vi "main002.vi"() -> ()   [LabVIEW 2019]
uses:
  <vilib>/DAQmx/write.llb/DAQmx Write (Analog DBL 1Chan 1Samp).vi
  <vilib>/DAQmx/miscellaneous.llb/DAQmx Fill In Error Info.vi
  <vilib>/DAQmx/create/channels.llb/DAQmx Create Channel (AO-Voltage-Basic).vi
  libs/Newport ESP301/Newport ESP301.lvlib
panel:
  in  "Boolean":bool
  out "a":waveform(dbl)(graph)={"t0"=timestamp(3633530059.5453157 s since 1904-01-01), "dt"=1.0, "Y"=[nan]}
  out "Waveform Chart":dbl(graph)=5.25341140860948
  out "x*y":dbl=nan
  in  "physical channels":tag="Dev3/ao1"
  out "DAC error":errorcluster
  out "ESP error":errorcluster={"status"=TRUE, "code"=-1074000000, "source"="Newport ESP301.lvlib:Error Query.vi<ERR>\nInstrument reports:\n313, 62119445, AXIS-3 MOTOR NOT ENABLED\r\n313, 62124900, AXIS-3 MOTOR NOT ENABLED\r\n313, 62130330, AXIS-3 MOTOR NOT ENABLED\r\n313, 62135785, AXIS-3 MOTOR NOT ENABLED\r\n313, 62141219, AXIS-3 MOTOR NOT ENABLED\r\n313, 62146768, AXIS-3 MOTOR NOT ENABLED\r\n313, 62152226, AXIS-3 MOTOR NOT ENABLED\r\n313, 62157684, AXIS-3 MOTOR NOT ENABLED\r\n313, 62163236, AXIS-3 MOTOR NOT ENABLED\r\n313, 62168690, AXIS-3 MOTOR NOT ENABLED\r\n0, 499821715, NO ERROR DETECTED\r\n\n\n\n<b>Complete call chain:</b>\r\n     Newport ESP301.lvlib:Error Query.vi\r\n     Newport ESP301.lvlib:Initialize.vi\r\n     main002.vi"}
  out "run?":bool
  in  "set_vel":bool
  in  "velocity [fs/s]":dbl=667.128190396304
  in  "vel_mm":dbl caption="velocity [mm/s]"
  out "meas. velocity":dbl=nan
  in  "stop":bool
  out "output voltage":dbl=nan
  in  "start":bool
  in  "go2p1":bool
  out "position [fs]":dbl=nan
  out "position [mm]":dbl=nan
  in  "p2 [mm]":dbl=2.0
  in  "p1 [mm]":dbl
  in  "interpolate output":bool
  in  "t2 [fs]":dbl=6671.281903963041
  in  "t1 [fs]":dbl=-6671.281903963041
  in  "t0 [mm]":dbl=1.0
  in  "Axis (1)":i32=3 min=1 max=3
  in  "Serial Link (RS232)":enum16{"RS232", "USB"}(ring)
  in  "VISA resource name":refnum<visa-resource-name>="COM9"
  in  "main_close":bool
  # "Always use CLOSE button to correctly disconnect the device. STOP program afterwards."
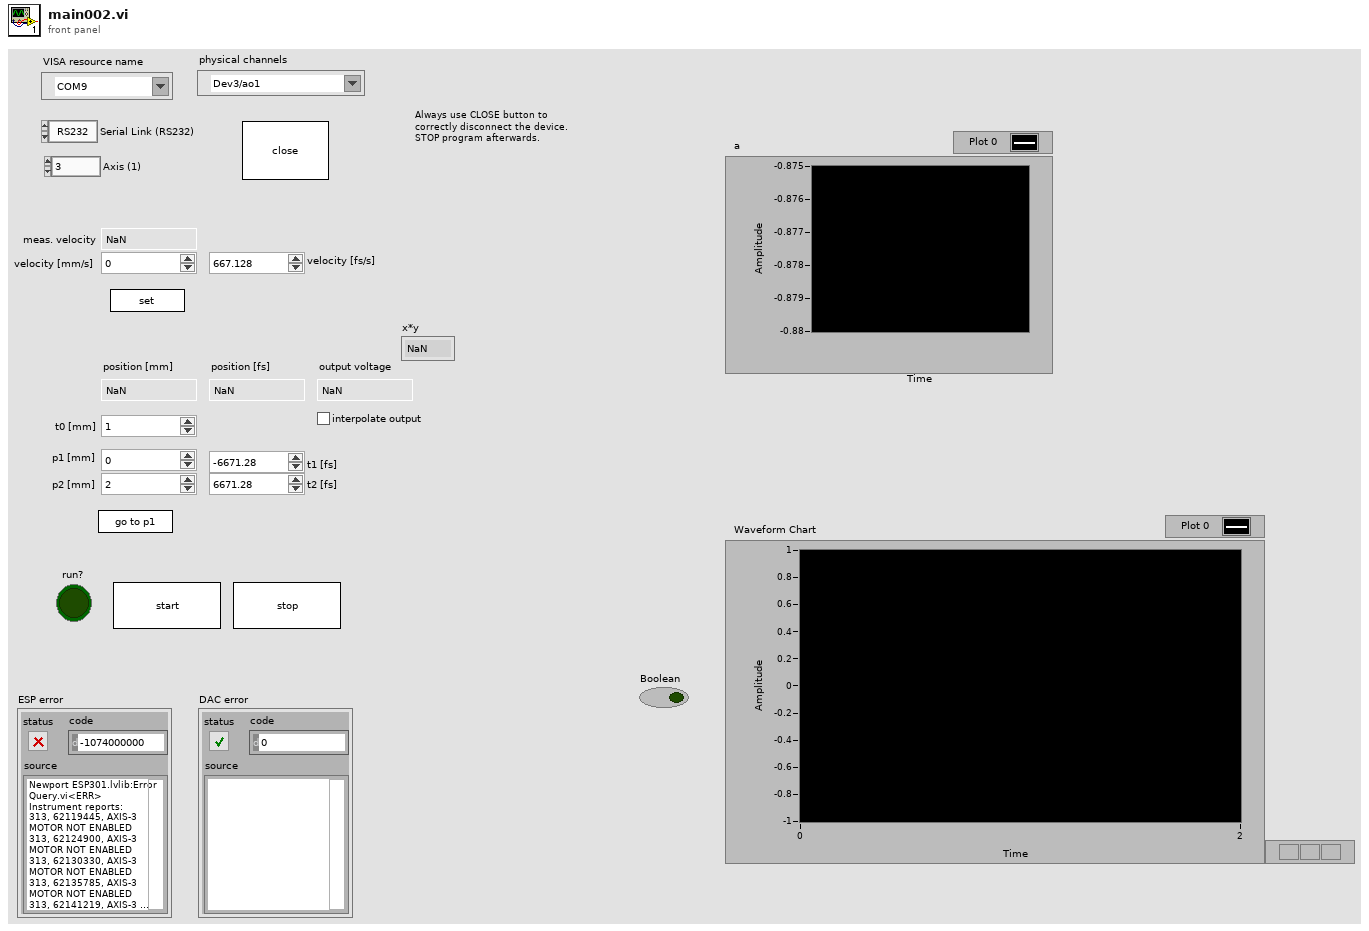
[diagram p1: front panel]
types:
  T1 = cluster{"dev1_data":refnum<queue>, "dev2_data":refnum<queue>}
  T2 = cluster{"dev1_cmd":refnum<queue>, "dev2_cmd":refnum<queue>}
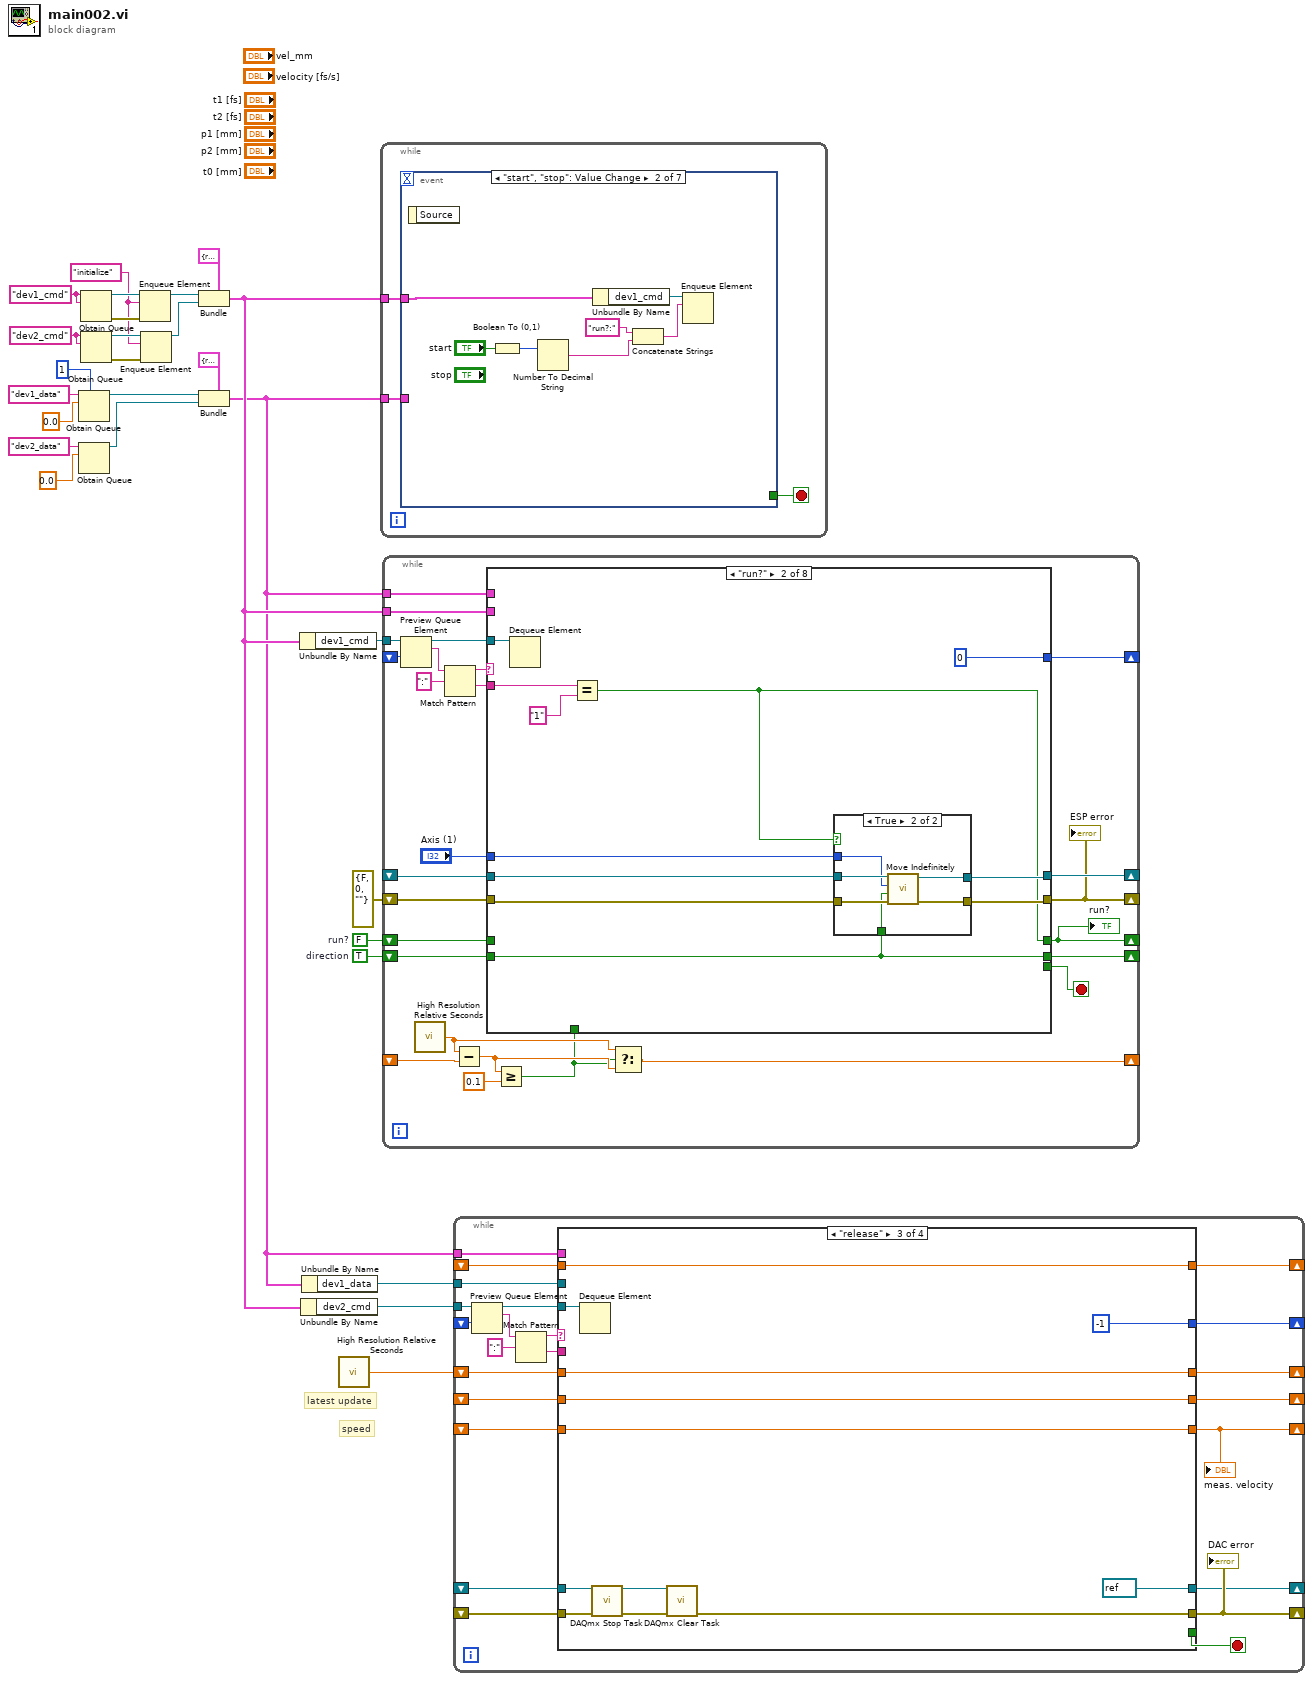
[diagram p0: block diagram]
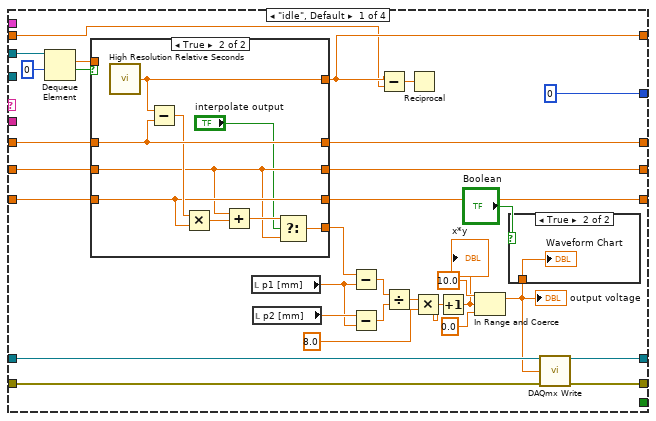
[diagram p2: hidden frame]
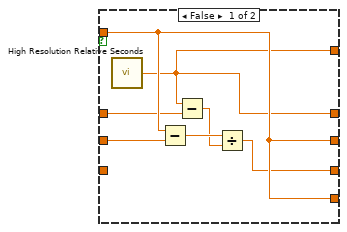
[diagram p4: hidden frame]
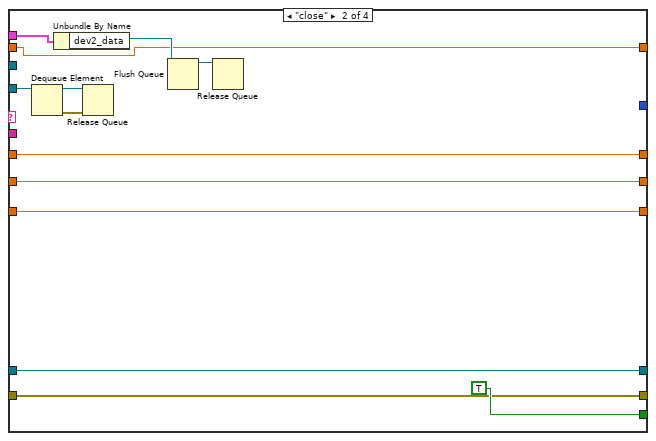
[diagram p5: hidden frame]
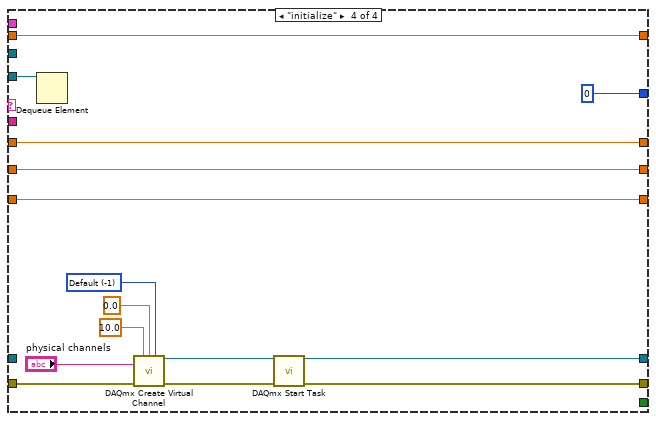
[diagram p6: hidden frame]
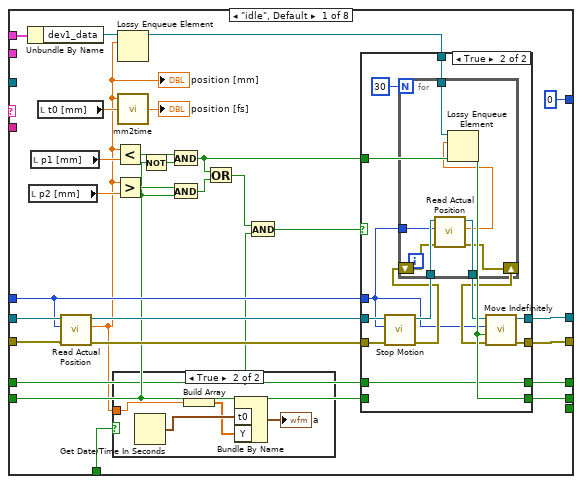
[diagram p7: hidden frame]
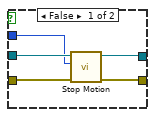
[diagram p10: hidden frame]
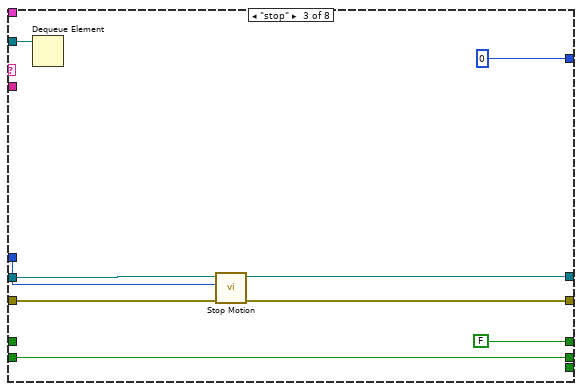
[diagram p11: hidden frame]
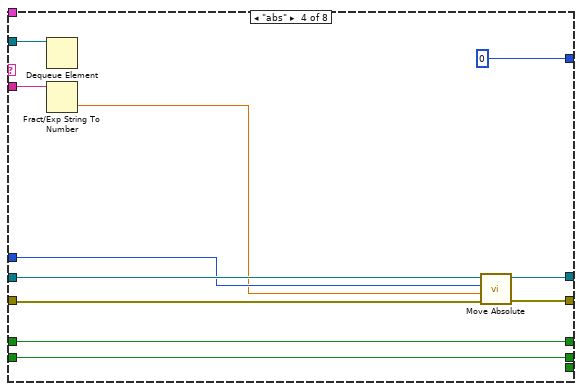
[diagram p12: hidden frame]
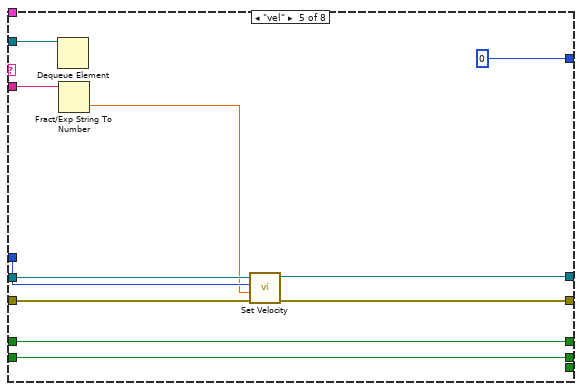
[diagram p13: hidden frame]
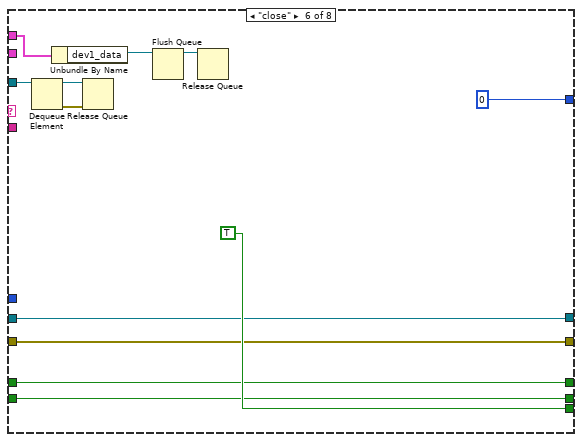
[diagram p14: hidden frame]
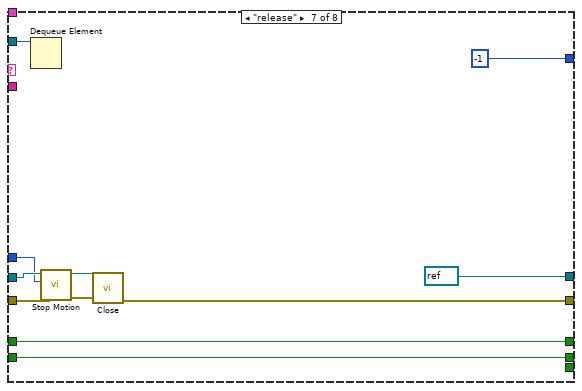
[diagram p15: hidden frame]
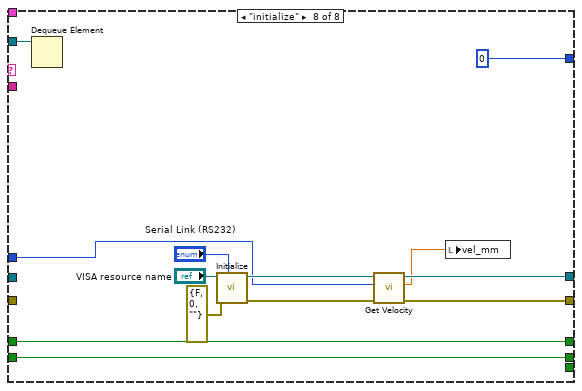
[diagram p16: hidden frame]
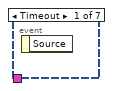
[diagram p17: hidden frame]
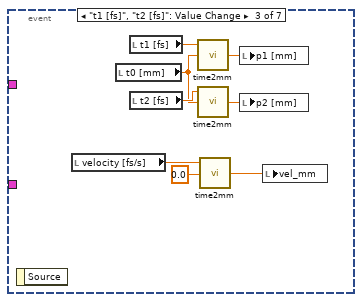
[diagram p18: hidden frame]
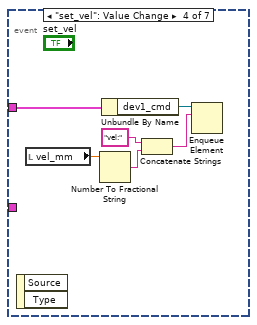
[diagram p19: hidden frame]
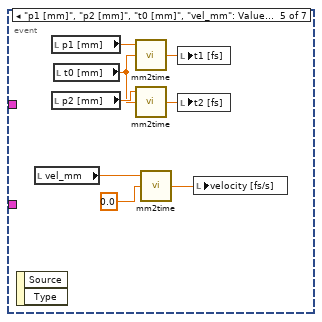
[diagram p20: hidden frame]
diagram:
  w1 = TRUE  # direction
  w4 = FALSE  # run?
  w15 = "dev2_cmd" ("name (unnamed)")
  w21 = "initialize" ("element")
  w16 = "dev1_cmd" ("name (unnamed)")
  # "speed"
  # "latest update"
  n1 = Obtain Queue(max queue size (-1, unlimited)=1, name (unnamed)="dev1_data", element data type=0.0) -> (queue out=w12:refnum<queue>)  [unwired: 2 in, 2 out]
  n2 = Obtain Queue(name (unnamed)="dev2_data", element data type=0.0) -> (queue out=w11:refnum<queue>)  [unwired: 3 in, 2 out]
  n3 = Obtain Queue(name (unnamed)=w16, element data type=w16) -> (queue out=w27:refnum<queue>, error out=w26:errorcluster)  [unwired: 3 in, 1 out]
  n4 = Obtain Queue(name (unnamed)=w15, element data type=w15) -> (queue out=w22:refnum<queue>, error out=w23:errorcluster)  [unwired: 3 in, 1 out]
  n5 = Enqueue Element(queue=w27, element=w21, error in (no error)=w26) -> (queue out=w24:refnum<queue>)  [unwired: 1 in, 2 out]
  n6 = Enqueue Element(queue=w22, element=w21, error in (no error)=w23) -> (queue out=w20:refnum<queue>)  [unwired: 1 in, 2 out]
  n7 = Bundle(cluster=T2 {"dev1_cmd"=refnum, "dev2_cmd"=refnum}, "dev1_cmd"=w24, "dev2_cmd"=w20) -> (w8:T2)
  n8 = Bundle(cluster=T1 {"dev1_data"=refnum, "dev2_data"=refnum}, "dev1_data"=w12, "dev2_data"=w11) -> (w2:T1)
  n9 = Unbundle By Name(w8) -> ("dev1_cmd"=w17:refnum<queue>)
  n10 = Unbundle By Name(w8) -> ("dev2_cmd"=w7:refnum<queue>)
  n11 = Unbundle By Name(w2) -> ("dev1_data"=w6:refnum<queue>)
  n12 = call <vilib>:"High Resolution Relative Seconds.vi"() -> ("relative seconds"=w5:dbl)
  n13 = while {
    tunnel: w8 -> [w30]
    tunnel: w2 -> [w29]
    stop <- w28 stop-if-true
    n14 = event shown="[1] \"start\", \"stop\": Value Change" {
      selector: _ -> [_ _ _ _ _ _ _]
      dyn-events: _ -> [_ _ _ _ _ _ _]
      timeout: _ -> [_ _ _ _ _ _ _]
      tunnel: w30 -> [_ w34 _ w47 _ w65 w68]
      tunnel: w29 -> [_ _ _ _ _ _ _]
      tunnel: [_ _ _ _ _ _ TRUE] -> w28
      event Timeout {
        n15 = event-data() -> ()  [unwired: 1 in, 1 out]
      }
      event "start", "stop": Value Change {
        n16 = event-data() -> ()  [unwired: 1 in, 1 out]
        n17 = Boolean To (0,1)(Boolean="start") -> (0, 1=w32:i16)
        n18 = Number To Decimal String(number=w32) -> (decimal integer string=w31:string)  [unwired: 1 in]
        n19 = Unbundle By Name(w34) -> ("dev1_cmd"=w37:refnum<queue>)
        n20 = Concatenate Strings("run?:" ("string"), w31) -> (w36:string)
        n21 = Enqueue Element(queue=w37, element=w36) -> ()  [unwired: 2 in, 3 out]
      }
      event "t1 [fs]", "t2 [fs]": Value Change {
        n22 = event-data() -> ()  [unwired: 1 in, 1 out]
        n23 = local read "velocity [fs/s]"() -> (w40:dbl)
        n24 = local read "t0 [mm]"() -> (w43:dbl)
        n25 = local read "t1 [fs]"() -> (w44:dbl)
        n26 = local read "t2 [fs]"() -> (w45:dbl)
        n27 = call "time2mm.vi"("Offset (mm)"=w43, "time"=w44) -> ("position (mm)"=w41:dbl)  [unwired: 1 in]
        n28 = call "time2mm.vi"("Offset (mm)"=w43, "time"=w45) -> ("position (mm)"=w42:dbl)  [unwired: 1 in]
        n29 = call "time2mm.vi"("Offset (mm)"=0.0, "time"=w40) -> ("position (mm)"=w38:dbl)  [unwired: 1 in]
        n30 = local write "p1 [mm]"(w41) -> ()
        n31 = local write "p2 [mm]"(w42) -> ()
        n32 = local write "vel_mm"(w38) -> ()
      }
      event "set_vel": Value Change {
        n33 = event-data() -> ()  [unwired: 1 in, 2 out]
        n34 = local read "vel_mm"() -> (w46:dbl)
        n35 = Number To Fractional String(number=w46) -> (F-format string=w50:string)  [unwired: 3 in]
        n36 = Unbundle By Name(w47) -> ("dev1_cmd"=w51:refnum<queue>)
        n37 = Concatenate Strings("vel:" ("string"), w50) -> (w49:string)
        n38 = Enqueue Element(queue=w51, element=w49) -> ()  [unwired: 2 in, 3 out]
      }
      event "p1 [mm]", "p2 [mm]", "t0 [mm]", "vel_mm": Value Change {
        n39 = event-data() -> ()  [unwired: 1 in, 2 out]
        n40 = local read "vel_mm"() -> (w54:dbl)
        n41 = local read "p1 [mm]"() -> (w58:dbl)
        n42 = local read "p2 [mm]"() -> (w59:dbl)
        n43 = local read "t0 [mm]"() -> (w57:dbl)
        n44 = call "mm2time.vi"("Offset (mm)"=w57, "distance (mm)"=w58) -> ("time in fs"=w55:dbl)  [unwired: 1 in]
        n45 = call "mm2time.vi"("Offset (mm)"=w57, "distance (mm)"=w59) -> ("time in fs"=w56:dbl)  [unwired: 1 in]
        n46 = call "mm2time.vi"("Offset (mm)"=0.0, "distance (mm)"=w54) -> ("time in fs"=w53:dbl)  [unwired: 1 in]
        n47 = local write "t1 [fs]"(w55) -> ()
        n48 = local write "t2 [fs]"(w56) -> ()
        n49 = local write "velocity [fs/s]"(w53) -> ()
      }
      event "go2p1": Value Change {
        n50 = event-data() -> ()  [unwired: 1 in, 2 out]
        n51 = local read "p1 [mm]"() -> (w60:dbl)
        n52 = Number To Fractional String(number=w60) -> (F-format string=w63:string)  [unwired: 3 in]
        n53 = Unbundle By Name(w65) -> ("dev1_cmd"=w64:refnum<queue>)
        n54 = Concatenate Strings("abs:" ("string"), w63) -> (w61:string)
        n55 = Enqueue Element(queue=w64, element=w61) -> ()  [unwired: 2 in, 3 out]
      }
      event "main_close": Value Change {
        n56 = event-data() -> ()  [unwired: 1 in, 1 out]
        n57 = Cluster To Array(cluster=w68) -> (array=w67:refnum<queue>[])
        n58 = for {
          tunnel: w67 -> [w73] mode=indexing
          n59 = Flush Queue(queue=w73) -> (queue out=w69:refnum<queue>)  [unwired: 1 in, 2 out]
          n60 = Enqueue Element(queue=w69, element="release") -> (queue out=w71:refnum<queue>)  [unwired: 2 in, 2 out]
          n61 = Enqueue Element(queue=w71, element="close") -> ()  [unwired: 2 in, 3 out]
        }
      }
    }
  }
  n62 = while {
    tunnel: w8 -> [w94]
    tunnel: w17 -> [w99]
    tunnel: w2 -> [w91]
    shift-right: [w89] -> _
    shift-left: _ -> [w90]
    shift-right: [w88] -> _
    shift-left: _ -> [w85]
    shift-right: [w87] -> _
    shift-left: errorcluster {"status"=FALSE, "code"=0, "source"=""} ("error out") -> [w86]
    shift-right: [w82] -> _
    shift-left: w4 -> [w83]
    shift-right: [w80] -> _
    shift-left: w1 -> [w81]
    shift-right: [w74] -> _
    shift-left: _ -> [w79]
    stop <- w92 stop-if-true
    n63 = Preview Queue Element(queue=w99, timeout in ms (-1)=w90) -> (queue out=w93:refnum<queue>, element=w98:string)  [unwired: 1 in, 2 out]
    n64 = call <vilib>:"High Resolution Relative Seconds.vi"() -> ("relative seconds"=w76:dbl)
    n65 = Match Pattern(string=w98, regular expression=":") -> (before substring=w96:string, after substring=w95:string)  [unwired: 1 in, 2 out]
    n66 = Subtract(x=w76, y=w79) -> (x-y=w77:dbl)
    n67 = Greater Or Equal?(x=w77, y=0.1) -> (x >= y?=w75:bool)
    n68 = case shown="\"run?\"" w96 {
      tunnel: w95 -> [_ w166 _ w196 w203 _ _ _]
      tunnel: w94 -> [_ _ _ _ _ _ _ _]
      tunnel: w93 -> [_ w164 w179 w197 w201 w220 w230 w240]
      tunnel: [_ _ _ _ _ TRUE _ _] -> w92
      tunnel: w91 -> [w126 _ _ _ _ w212 _ _]
      tunnel: [0 0 0 0 0 0 -1 0] -> w89
      tunnel: [w122 w161 w184 w193 w208 w216 refnum<visa-resource-name> refnum ("VISA resource name out") w236] -> w88
      tunnel: [w121 w160 w183 w192 w207 w215 w229 w235] -> w87
      tunnel: w86 -> [w117 w158 w185 w194 w206 w215 w225 _]
      tunnel: w85 -> [w119 w159 w186 w195 w205 w216 w222 _]
      tunnel: "Axis (1)" -> [w118 w162 w182 w191 w204 _ w221 w237]
      tunnel: w83 -> [w104 _ _ w188 w199 w213 w227 w241]
      tunnel: [w103 w157 FALSE ("run?") w188 w199 w213 w227 w241] -> w82
      tunnel: w81 -> [w105 w156 w178 w187 w198 w209 w226 w232]
      tunnel: [w106 w156 w178 w187 w198 w209 w226 w232] -> w80
      tunnel: w75 -> [w102 _ _ _ _ _ _ _]
      frame "idle", Default {
        n69 = Unbundle By Name(w126) -> ("dev1_data"=w125:refnum<queue>)
        n70 = local read "p2 [mm]"() -> (w113:dbl)
        n71 = local read "p1 [mm]"() -> (w114:dbl)
        n72 = local read "t0 [mm]"() -> (w124:dbl)
        n73 = call "Read Actual Position.vi"("error in (no error)"=w117, "Axis (1)"=w118, "VISA resource name"=w119) -> ("error out"=w116:errorcluster, "Position (units)"=w101:dbl, "VISA resource name out"=w115:refnum<visa-resource-name>)  [unwired: 2 in]
        "position [mm]" <- w101
        n74 = case shown="True" w102 {
          tunnel: w101 -> [_ w131]
          frame False {
          }
          frame True {
            n75 = Get Date/Time In Seconds() -> (seconds since 1Jan1904=w130:timestamp)
            n76 = Build Array(w131) -> (w129:dbl[])
            n77 = Bundle By Name("t0"=w130, "Y"=w129) -> (→"a":waveform(dbl))  [unwired: 1 in]
          }
        }
        n78 = Less?(x=w101, y=w114) -> (x < y?=w111:bool)
        n79 = Greater?(x=w101, y=w113) -> (0:w110:bool)
        n80 = Lossy Enqueue Element(queue=w125, element=w101) -> (queue out=w100:refnum<queue>)  [unwired: 1 in, 3 out]
        n81 = call "mm2time.vi"("Offset (mm)"=w124, "distance (mm)"=w101) -> ("time in fs"=→"position [fs]":dbl)  [unwired: 1 in]
        n82 = Not(x=w105) -> (.not. x?=w112:bool)
        n83 = And(x=w111, y=w112) -> (x .and. y?=w107:bool)
        n84 = And(x=w110, y=w105) -> (x .and. y?=w109:bool)
        n85 = Or(x=w107, y=w109) -> (x .or. y?=w108:bool)
        n86 = And(x=w108, y=w104) -> (x .and. y?=w120:bool)
        n87 = case shown="True" w120 {
          tunnel: w115 -> [w135 w146]
          tunnel: w116 -> [w134 w145]
          tunnel: [w135 w148] -> w122
          tunnel: [w134 w147] -> w121
          tunnel: w118 -> [_ w138]
          tunnel: w107 -> [_ w144]
          tunnel: [w133 w144] -> w106
          tunnel: w105 -> [w133 _]
          tunnel: w104 -> [w132 w143]
          tunnel: [w132 w143] -> w103
          tunnel: w100 -> [_ w137]
          frame False {
          }
          frame True {
            n88 = call "Stop Motion.vi"("error in (no error)"=w145, "Axis (1)"=w138, "VISA resource name"=w146) -> ("error out"=w140:errorcluster, "VISA resource name out"=w142:refnum<visa-resource-name>)  [unwired: 3 in]
            n89 = for {
              N: 30 -> [_]
              tunnel: w142 -> [w155]
              tunnel: [w154] -> w141
              shift-right: [w152] -> w139
              shift-left: w140 -> [w153]
              tunnel: w138 -> [w151]
              tunnel: w137 -> [w150]
              n90 = call "Read Actual Position.vi"("error in (no error)"=w153, "Axis (1)"=w151, "VISA resource name"=w155) -> ("error out"=w152:errorcluster, "Position (units)"=w149:dbl, "VISA resource name out"=w154:refnum<visa-resource-name>)  [unwired: 2 in]
              n91 = Lossy Enqueue Element(queue=w150, element=w149) -> ()  [unwired: 1 in, 4 out]
            }
            n92 = call "Move Indefinitely.vi"("error in (no error)"=w139, "Move Direction (+)"=w144, "Axis (1)"=w138, "VISA resource name"=w141) -> ("error out"=w147:errorcluster, "VISA resource name out"=w148:refnum<visa-resource-name>)  [unwired: 2 in]
          }
        }
      }
      frame "run?" {
        n93 = Dequeue Element(queue=w164) -> ()  [unwired: 2 in, 4 out]
        n94 = Equal?(x=w166, y="1") -> (x = y?=w157:bool)
        n95 = case shown="True" w157 {
          tunnel: w159 -> [w171 w177]
          tunnel: w158 -> [w168 w176]
          tunnel: w162 -> [w167 w175]
          tunnel: [w170 w174] -> w161
          tunnel: [w169 w173] -> w160
          tunnel: w156 -> [_ w172]
          frame False {
            n96 = call "Stop Motion.vi"("error in (no error)"=w168, "Axis (1)"=w167, "VISA resource name"=w171) -> ("error out"=w169:errorcluster, "VISA resource name out"=w170:refnum<visa-resource-name>)  [unwired: 3 in]
          }
          frame True {
            n97 = call "Move Indefinitely.vi"("error in (no error)"=w176, "Move Direction (+)"=w172, "Axis (1)"=w175, "VISA resource name"=w177) -> ("error out"=w173:errorcluster, "VISA resource name out"=w174:refnum<visa-resource-name>)  [unwired: 2 in]
          }
        }
      }
      frame "stop" {
        n98 = Dequeue Element(queue=w179) -> ()  [unwired: 2 in, 4 out]
        n99 = call "Stop Motion.vi"("error in (no error)"=w185, "Axis (1)"=w182, "VISA resource name"=w186) -> ("error out"=w183:errorcluster, "VISA resource name out"=w184:refnum<visa-resource-name>)  [unwired: 3 in]
      }
      frame "abs" {
        n100 = Dequeue Element(queue=w197) -> ()  [unwired: 2 in, 4 out]
        n101 = Fract/Exp String To Number(string=w196) -> (number=w190:dbl)  [unwired: 3 in, 1 out]
        n102 = call "Move Absolute.vi"("error in (no error)"=w194, "Position (0 units)"=w190, "Axis (1)"=w191, "VISA resource name"=w195) -> ("error out"=w192:errorcluster, "VISA resource name out"=w193:refnum<visa-resource-name>)  [unwired: 2 in]
      }
      frame "vel" {
        n103 = Dequeue Element(queue=w201) -> ()  [unwired: 2 in, 4 out]
        n104 = Fract/Exp String To Number(string=w203) -> (number=w202:dbl)  [unwired: 3 in, 1 out]
        n105 = call "Set Velocity.vi"("error in (no error)"=w206, "Velocity (units/s)"=w202, "Axis (1)"=w204, "VISA resource name"=w205) -> ("error out"=w207:errorcluster, "VISA resource name out"=w208:refnum<visa-resource-name>)  [unwired: 2 in]
      }
      frame "close" {
        n106 = Dequeue Element(queue=w220) -> (queue out=w219:refnum<queue>, error out=w218:errorcluster)  [unwired: 2 in, 2 out]
        n107 = Unbundle By Name(w212) -> ("dev1_data"=w210:refnum<queue>)
        n108 = Release Queue(queue=w219, error in (no error)=w218) -> ()  [unwired: 1 in, 3 out]
        n109 = Flush Queue(queue=w210) -> (queue out=w211:refnum<queue>)  [unwired: 1 in, 2 out]
        n110 = Release Queue(queue=w211) -> ()  [unwired: 2 in, 3 out]
      }
      frame "release" {
        n111 = Dequeue Element(queue=w230) -> ()  [unwired: 2 in, 4 out]
        n112 = call "Stop Motion.vi"("error in (no error)"=w225, "Axis (1)"=w221, "VISA resource name"=w222) -> ("error out"=w224:errorcluster, "VISA resource name out"=w223:refnum<visa-resource-name>)  [unwired: 3 in]
        n113 = call "Close.vi"("error in (no error)"=w224, "VISA resource name"=w223) -> ("error out"=w229:errorcluster)  [unwired: 9 in]
      }
      frame "initialize" {
        n114 = Dequeue Element(queue=w240) -> ()  [unwired: 2 in, 4 out]
        n115 = call "Initialize.vi"("VISA resource name"="VISA resource name", "error in (no error)"=errorcluster {"status"=FALSE, "code"=0, "source"=""}, "Serial Link (RS232)"="Serial Link (RS232)") -> ("VISA resource name out"=w239:refnum<visa-resource-name>, "error out"=w238:errorcluster)  [unwired: 6 in]
        n116 = call "Get Velocity.vi"("error in (no error)"=w238, "Axis (1)"=w237, "VISA resource name"=w239) -> ("error out"=w235:errorcluster, "Velocity (units/s)"=w234:dbl, "VISA resource name out"=w236:refnum<visa-resource-name>)  [unwired: 2 in]
        n117 = local write "vel_mm"(w234) -> ()
      }
    }
    "run?" <- w82
    "ESP error" <- w87
    n118 = Select(t=w76, s=w75, f=w77) -> (s? t:f=w74:dbl)
  }
  n119 = while {
    shift-right: [w260] -> _
    shift-left: _ -> [w261]
    shift-right: [w259] -> _
    shift-left: _ -> [w258]
    tunnel: w7 -> [w257]
    shift-right: [w256] -> _
    shift-left: _ -> [w255]
    tunnel: w6 -> [w254]
    shift-right: [w253] -> _
    shift-left: _ -> [w250]
    shift-right: [w252] -> _
    shift-left: w5 -> [w251]
    shift-right: [w245] -> _
    shift-left: _ -> [w249]
    tunnel: w2 -> [w248]
    shift-right: [w247] -> _
    shift-left: _ -> [w246]
    stop <- w262 stop-if-true
    n120 = Preview Queue Element(queue=w257, timeout in ms (-1)=w261) -> (queue out=w263:refnum<queue>, element=w267:string)  [unwired: 1 in, 2 out]
    n121 = Match Pattern(string=w267, regular expression=":") -> (before substring=w265:string, after substring=w264:string)  [unwired: 1 in, 2 out]
    n122 = case shown="\"release\"" w265 {
      tunnel: w264 -> [_ _ _ _]
      tunnel: w263 -> [_ w328 w339 w347]
      tunnel: [_ TRUE _ _] -> w262
      tunnel: [0 _ -1 0] -> w260
      tunnel: [w294 w324 w338 w348] -> w259
      tunnel: w258 -> [w292 w324 w335 w355]
      tunnel: [w295 w323 refnum<k21> refnum ("task out") w349] -> w256
      tunnel: w255 -> [w293 w323 w336 _]
      tunnel: w254 -> [w296 _ _ _]
      tunnel: [w290 w321 w331 w344] -> w253
      tunnel: [w289 w322 w332 w345] -> w252
      tunnel: w251 -> [w287 w322 w332 w345]
      tunnel: w250 -> [w288 w321 w331 w344]
      tunnel: [w286 w320 w330 w343] -> w245
      tunnel: w249 -> [w285 w320 w330 w343]
      tunnel: w248 -> [_ w317 _ _]
      tunnel: [w274 w316 w329 w341] -> w247
      tunnel: w246 -> [w273 w316 w329 w341]
      frame "idle", Default {
        n123 = Dequeue Element(queue=w296, timeout in ms (-1)=0) -> (element=w291:dbl, timed out?=w275:bool)  [unwired: 1 in, 2 out]
        n124 = case shown="True" w275 {
          tunnel: w291 -> [w306 _]
          tunnel: [w306 w308] -> w284
          tunnel: [w306 w310] -> w290
          tunnel: [w300 w315] -> w289
          tunnel: w288 -> [w305 w310]
          tunnel: w287 -> [w304 w315]
          tunnel: [w301 w312] -> w286
          tunnel: w285 -> [_ w312]
          tunnel: [w300 w307] -> w274
          frame False {
            n125 = call <vilib>:"High Resolution Relative Seconds.vi"() -> ("relative seconds"=w300:dbl)
            n126 = Subtract(x=w306, y=w305) -> (x-y=w303:dbl)
            n127 = Subtract(x=w300, y=w304) -> (x-y=w302:dbl)
            n128 = Divide(x=w303, y=w302) -> (x/y=w301:dbl)
          }
          frame True {
            n129 = call <vilib>:"High Resolution Relative Seconds.vi"() -> ("relative seconds"=w307:dbl)
            n130 = Subtract(x=w307, y=w315) -> (x-y=w314:dbl)
            n131 = Multiply(x=w314, y=w312) -> (x*y=w313:dbl)
            n132 = Add(x=w310, y=w313) -> (x+y=w311:dbl)
            n133 = Select(t=w311, s="interpolate output", f=w310) -> (s? t:f=w308:dbl)
          }
        }
        n134 = local read "p1 [mm]"() -> (w282:dbl)
        n135 = local read "p2 [mm]"() -> (w283:dbl)
        n136 = Subtract(x=w284, y=w282) -> (x-y=w281:dbl)
        n137 = Subtract(x=w283, y=w282) -> (x-y=w280:dbl)
        n138 = Subtract(x=w274, y=w273) -> (x-y=w272:dbl)
        n139 = Divide(x=w281, y=w280) -> (x/y=w279:dbl)
        n140 = Reciprocal(x=w272) -> ()  [unwired: 1 out]
        n141 = Multiply(x=w279, y=8.0) -> (x*y=w270:dbl)
        n142 = Increment(x=w270) -> (x+1=w269:dbl)
        "x*y" <- w269
        n143 = In Range and Coerce(upper limit=10.0, x=w269, lower limit=0.0) -> (coerced(x)=w271:dbl)  [unwired: 1 out]
        "output voltage" <- w271
        n144 = case shown="True" "Boolean" {
          tunnel: w271 -> [_ w299]
          frame False {
          }
          frame True {
            "Waveform Chart" <- w299
          }
        }
        n145 = call-poly <vilib>:"DAQmx Write.vi"("task/channels in"=w293, "data"=w271, "error in"=w292) -> ("task out"=w295:refnum<k21>, "error out"=w294:errorcluster)  [unwired: 10 in, 1 out]
      }
      frame "close" {
        n146 = Dequeue Element(queue=w328) -> (queue out=w327:refnum<queue>, error out=w326:errorcluster)  [unwired: 2 in, 2 out]
        n147 = Unbundle By Name(w317) -> ("dev2_data"=w318:refnum<queue>)
        n148 = Release Queue(queue=w327, error in (no error)=w326) -> ()  [unwired: 1 in, 3 out]
        n149 = Flush Queue(queue=w318) -> (queue out=w319:refnum<queue>)  [unwired: 1 in, 2 out]
        n150 = Release Queue(queue=w319) -> ()  [unwired: 2 in, 3 out]
      }
      frame "release" {
        n151 = Dequeue Element(queue=w339) -> ()  [unwired: 2 in, 4 out]
        n152 = call <vilib>:"DAQmx Stop Task.vi"("task/channels in"=w336, "error in"=w335) -> ("task out"=w334:refnum<k21>, "error out"=w333:errorcluster)  [unwired: 12 in]
        n153 = call <vilib>:"DAQmx Clear Task.vi"("task in"=w334, "error in"=w333) -> ("error out"=w338:errorcluster)  [unwired: 13 in]
      }
      frame "initialize" {
        w352 = -1 items=["Default"=-1, "RSE"=10083, "Differential"=10106, "Pseudodifferential"=12529] ("output terminal configuration")
        n154 = Dequeue Element(queue=w347) -> ()  [unwired: 2 in, 4 out]
        n155 = call-poly <vilib>:"DAQmx Create Virtual Channel.vi"("maximum value"=10.0, "minimum value"=0.0, "output terminal configuration"=w352, "physical channels"="physical channels", "error in"=w355) -> ("task out"=w351:refnum<k21>, "error out"=w350:errorcluster)  [unwired: 9 in]
        n156 = call <vilib>:"DAQmx Start Task.vi"("task/channels in"=w351, "error in"=w350) -> ("task out"=w349:refnum<k21>, "error out"=w348:errorcluster)  [unwired: 12 in]
      }
    }
    "meas. velocity" <- w245
    "DAC error" <- w259
  }
